vi "set_continuous_volume_scan_flag.vi"(8 "error in (no error)":errorcluster, 10 "continuous volume scan?":bool, 11 "ImagingModeDL090130Frame in":refnum<class "ImagingModeDL090130Frame.lvclass">) -> (0 "error out":errorcluster, 3 "ImagingModeDL090130Frame out":refnum<class "ImagingModeDL090130Frame.lvclass">)   [LabVIEW 2010, in "ImagingModeDL090130Frame.lvclass"]
uses:
  ImagingModeDL090130Frame.lvclass
  ImagingModeDL090130Frame.lvclass/ImagingModeDL090130Frame.ctl
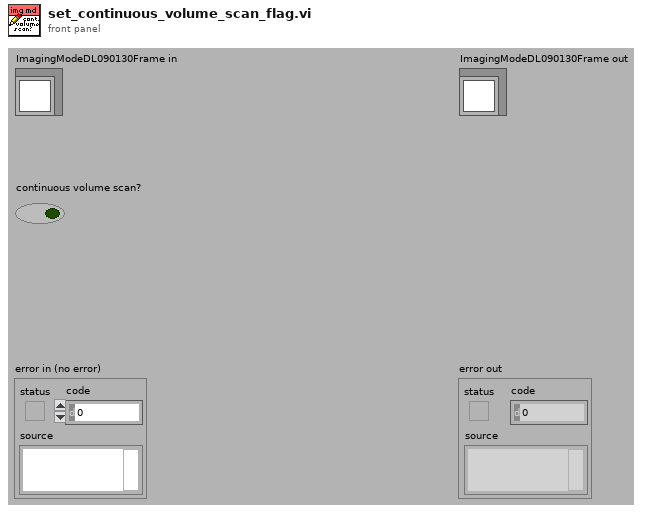
[diagram p1: front panel]
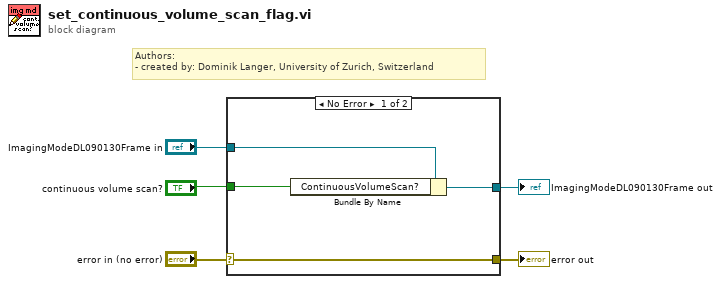
[diagram p0: block diagram]
diagram:
  # "Authors: \n- created by: Dominik Langer, University of Zurich, Switzerland"
  n1 = case shown="No Error" "error in (no error)" {
    selector: "error in (no error)" -> [w9 w11]
    tunnel: [w9 w11] -> w4
    tunnel: [w6 w10] -> w2
    tunnel: "ImagingModeDL090130Frame in" -> [w7 w10]
    tunnel: "continuous volume scan?" -> [w8 _]
    frame No Error {
      n2 = Bundle By Name(cluster=w7, "ContinuousVolumeScan?"=w8) -> (w6:refnum<class "ImagingModeDL090130Frame.lvclass">)
    }
    frame Error {
    }
  }
  "error out" <- w4
  "ImagingModeDL090130Frame out" <- w2
